vi "Read Value.vi"(8 "error in (no error)":errorcluster, 11 "WriteDigital in":refnum<class "WriteDigital.lvclass">) -> (0 "error out":errorcluster, 2 "Value":u16, 3 "WriteDigital out":refnum<class "WriteDigital.lvclass">)   [LabVIEW 2013, in "MaterialCharacterization.lvlib" / "WriteDigital.lvclass"]
uses:
  WriteDigital.lvclass
  WriteDigital.lvclass/WriteDigital.ctl
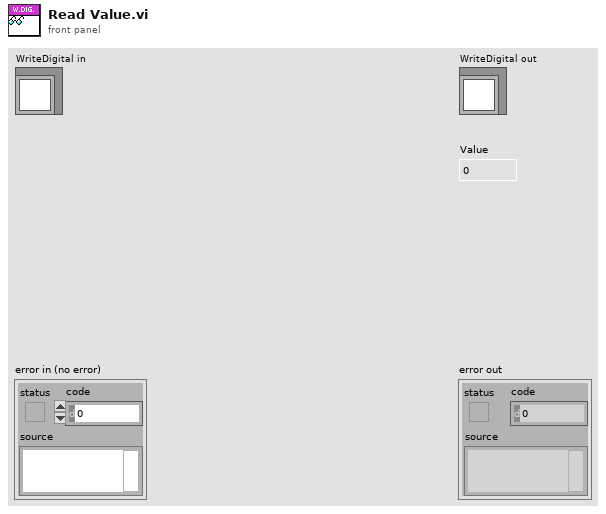
[diagram p1: front panel]
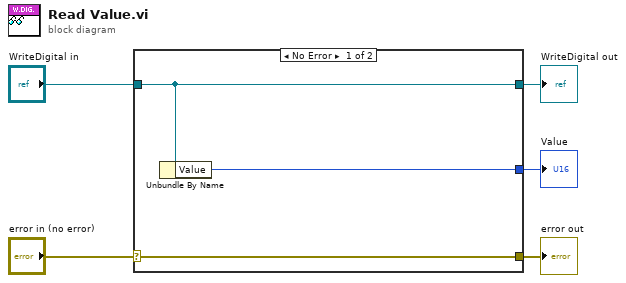
[diagram p0: block diagram]
diagram:
  n1 = case shown="No Error" "error in (no error)" {
    selector: "error in (no error)" -> [w8 w9]
    tunnel: [w8 w9] -> w4
    tunnel: [w7 w10] -> w2
    tunnel: "WriteDigital in" -> [w7 w10]
    tunnel: [w6 _] -> w1
    frame No Error {
      n2 = Unbundle By Name(w7) -> ("Value"=w6:u16)
    }
    frame Error {
    }
  }
  "error out" <- w4
  "WriteDigital out" <- w2
  "Value" <- w1
